vi "多参15分钟延时启动.vi"   [LabVIEW 2016]
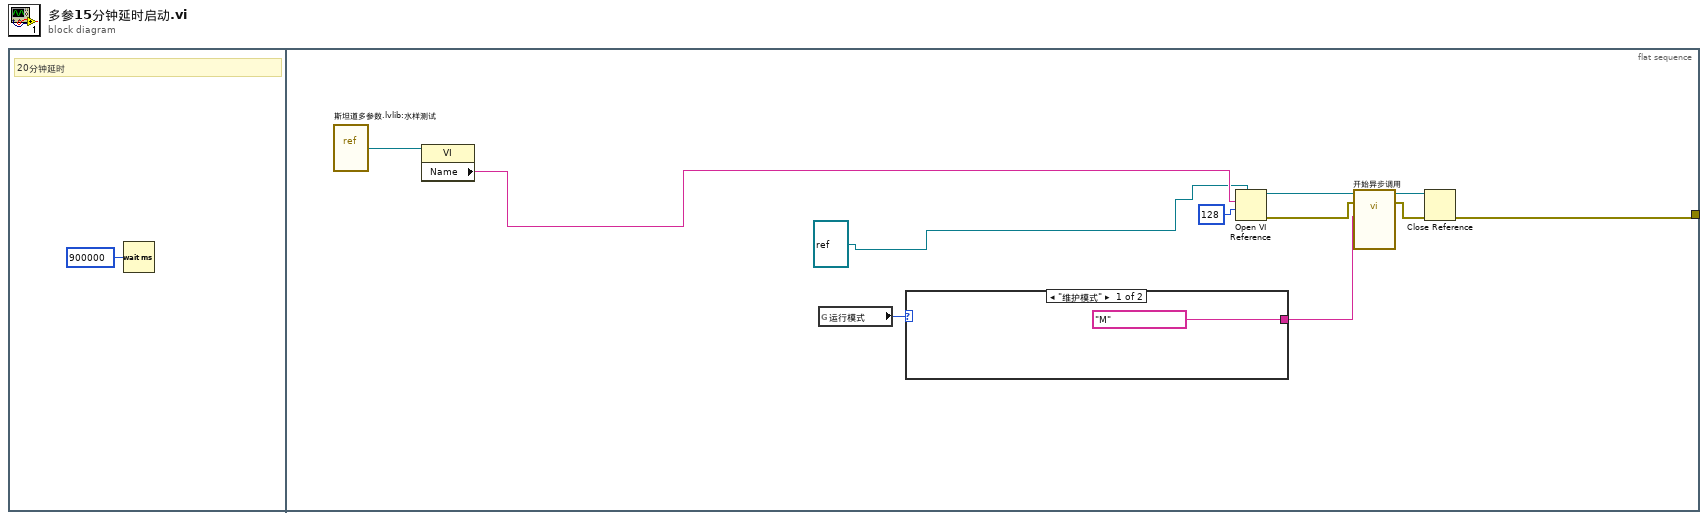
[diagram p0: block diagram]
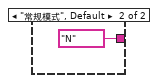
[diagram p2: hidden frame]
diagram:
  n1 = flat-sequence {
    tunnel: [w3] -> _
    frame #0 {
      # "20分钟延时"
      n2 = Wait (ms)(milliseconds to wait=u32 900000 ("等待时间（毫秒）")) -> ()  [unwired: 1 out]
    }
    frame #1 {
      n3 = vi-ref "斯坦道多参数.lvlib:水样测试.vi"() -> (w12:refnum<vi>)
      n4 = property class="VI"(reference=w12) -> ("Name"=w11:string)  [unwired: 1 in, 2 out]
      n5 = global read "系统设置全局变量.vi" "运行模式"() -> (w7:enum16{"维护模式", "常规模式", "应急模式", "质控模式"})
      n6 = case shown="\"维护模式\"" w7 {
        tunnel: ["M" ("数据标记表") "N" ("数据标记表")] -> w6
        frame "维护模式" {
        }
        frame "常规模式", Default {
        }
      }
      n7 = Open VI Reference(type specifier VI Refnum (for type only)=refnum<vi> refnum, vi path=w11, options=128 ("选项")) -> (vi reference=w9:refnum<vi>, error out=w2:errorcluster)  [unwired: 3 in]
      n8 = call-by-ref "开始异步调用"(reference=w9, error in=w2, "数据标记表"=w6) -> (reference out=w8:refnum<vi>, error out=w4:errorcluster)  [unwired: 11 in]
      n9 = Close Reference(reference=w8, error in (no error)=w4) -> (error out=w3:errorcluster)
    }
  }
